vi "Convert Package Attribute Cluster to String.vi"(8 "error in (no error)":errorcluster, 10 "package attributes":T1, 11 "initial package attributes string":string) -> (0 "error out":errorcluster, 3 "package attributes string out":string)   [LabVIEW 2014, in "NIPM_API.lvlib"]
uses:
  NIPM_API.lvlib
  package attributes.ctl
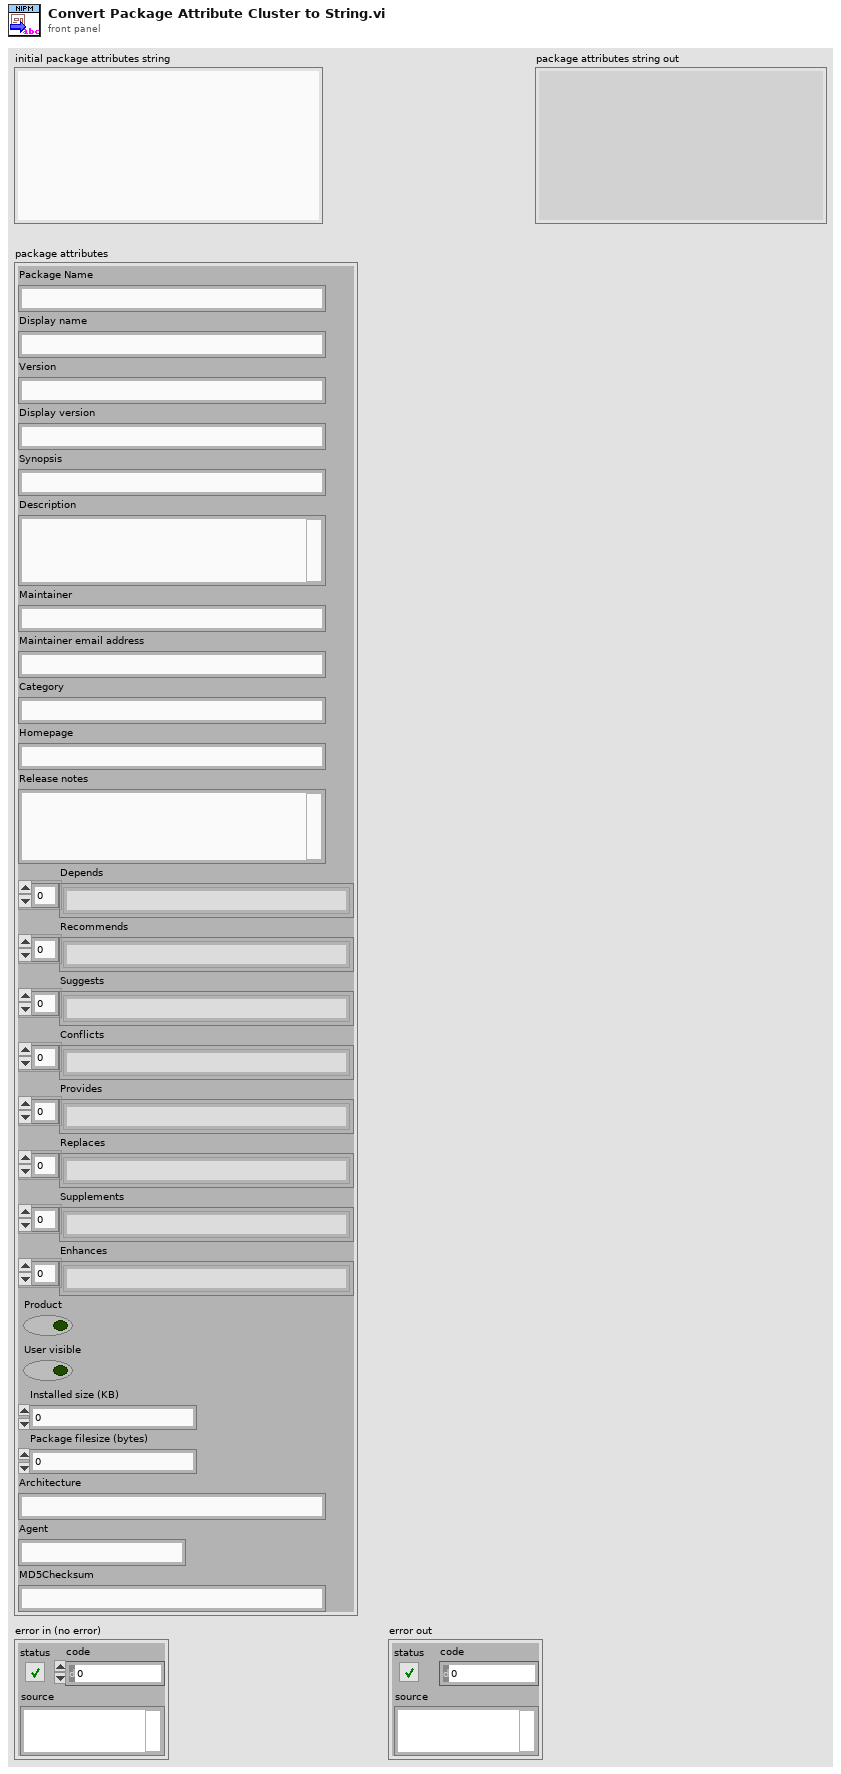
[diagram p1: front panel]
types:
  T1 = typedef "NIPM_API.lvlib/package attributes.ctl" = cluster{"Package Name":string, "Display name":string, "Version":string, "Display version":string, "Synopsis":string, "Description":string, "Maintainer":string, "Maintainer email address":string, "Category":string, "Homepage":string, "Release notes":string, "Depends":string[], "Recommends":string[], "Suggests":string[], "Conflicts":string[], "Provides":string[], "Replaces":string[], "Supplements":string[], "Enhances":string[], "Product":bool, "User visible":bool, "Installed size (KB)":u64, "Package filesize (bytes)":u64, "Architecture":string, "Agent":string, "MD5Checksum":string}
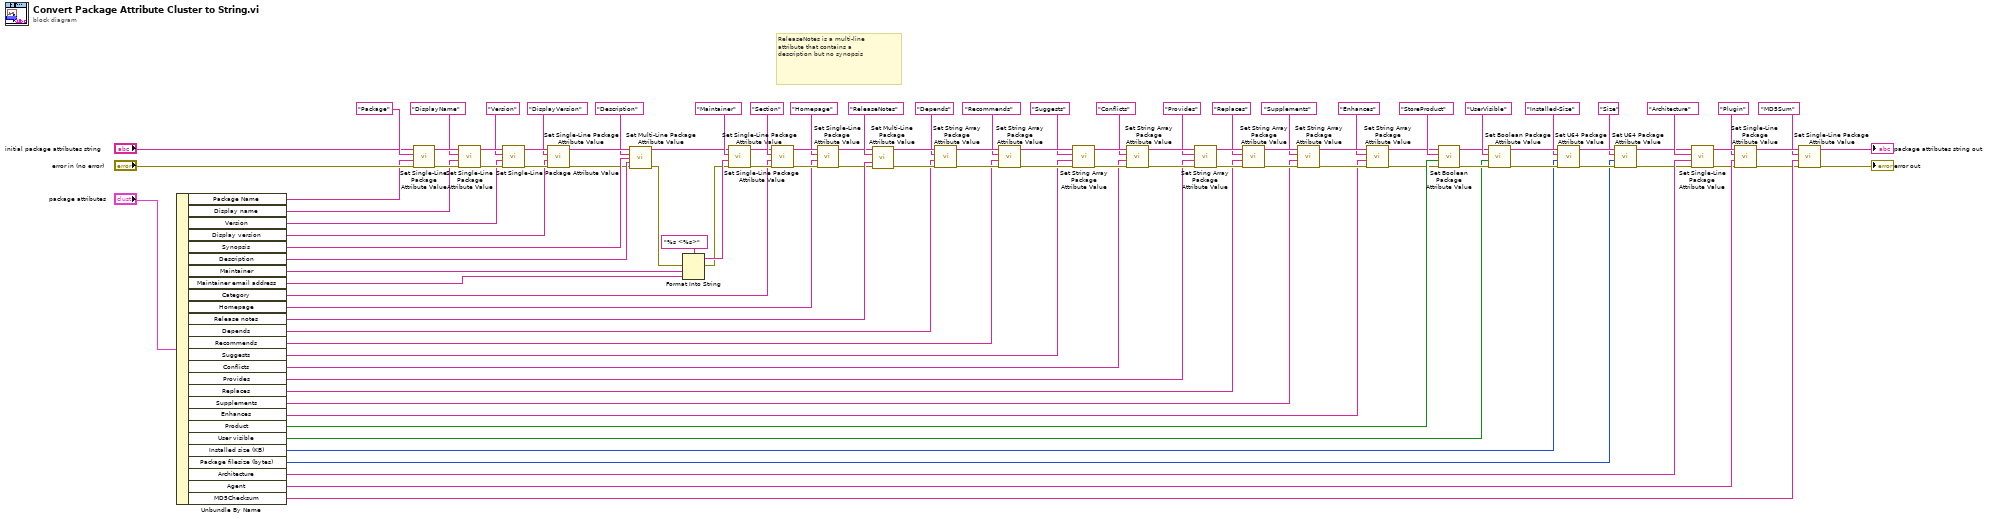
[diagram p0: block diagram]
diagram:
  # "ReleaseNotes is a multi-line attribute that contains a description but no synopsis"
  n1 = Unbundle By Name("package attributes") -> ("Package Name"=w91:string, "Display name"=w90:string, "Version"=w89:string, "Display version"=w88:string, "Synopsis"=w53:string, "Description"=w52:string, "Maintainer"=w69:string, "Maintainer email address"=w68:string, "Category"=w75:string, "Homepage"=w74:string, "Release notes"=w50:string, "Depends"=w20:string[], "Recommends"=w19:string[], "Suggests"=w18:string[], "Conflicts"=w17:string[], "Provides"=w16:string[], "Replaces"=w15:string[], "Supplements"=w14:string[], "Enhances"=w13:string[], "Product"=w60:bool, "User visible"=w59:bool, "Installed size (KB)"=w4:u64, "Package filesize (bytes)"=w3:u64, "Architecture"=w73:string, "Agent"=w72:string, "MD5Checksum"=w71:string)
  n2 = call "Set Single-Line Package Attribute Value.vi"("error in (no error)"="error in (no error)", "package attribute value"=w91, "package attribute name"="Package", "package attributes string in"="initial package attributes string") -> ("error out"=w97:errorcluster, "package attributes string out"=w100:string)  [unwired: 4 in, 2 out]
  n3 = call "Set Single-Line Package Attribute Value.vi"("error in (no error)"=w97, "package attribute value"=w90, "package attribute name"="DisplayName", "package attributes string in"=w100) -> ("error out"=w96:errorcluster, "package attributes string out"=w99:string)  [unwired: 4 in, 2 out]
  n4 = call "Set Single-Line Package Attribute Value.vi"("error in (no error)"=w96, "package attribute value"=w89, "package attribute name"="Version", "package attributes string in"=w99) -> ("error out"=w95:errorcluster, "package attributes string out"=w98:string)  [unwired: 4 in, 2 out]
  n5 = call "Set Single-Line Package Attribute Value.vi"("error in (no error)"=w95, "package attribute value"=w88, "package attribute name"="DisplayVersion", "package attributes string in"=w98) -> ("error out"=w51:errorcluster, "package attributes string out"=w56:string)  [unwired: 4 in, 2 out]
  n6 = call "Set Multi-Line Package Attribute Value.vi"("package attributes string in"=w56, "package attribute name"="Description", "synopsis"=w53, "description"=w52, "error in (no error)"=w51) -> ("package attributes string out"=w55:string, "error out"=w2:errorcluster)  [unwired: 7 in, 2 out]
  n7 = Format Into String(format string="%s <%s>", error in=w2, w69, w68) -> (resulting string=w70:string, error out=w1:errorcluster)  [unwired: 1 in]
  n8 = call "Set Single-Line Package Attribute Value.vi"("error in (no error)"=w1, "package attribute value"=w70, "package attribute name"="Maintainer", "package attributes string in"=w55) -> ("error out"=w82:errorcluster, "package attributes string out"=w85:string)  [unwired: 4 in, 2 out]
  n9 = call "Set Single-Line Package Attribute Value.vi"("error in (no error)"=w82, "package attribute value"=w75, "package attribute name"="Section", "package attributes string in"=w85) -> ("error out"=w81:errorcluster, "package attributes string out"=w84:string)  [unwired: 4 in, 2 out]
  n10 = call "Set Single-Line Package Attribute Value.vi"("error in (no error)"=w81, "package attribute value"=w74, "package attribute name"="Homepage", "package attributes string in"=w84) -> ("error out"=w49:errorcluster, "package attributes string out"=w47:string)  [unwired: 4 in, 2 out]
  n11 = call "Set Multi-Line Package Attribute Value.vi"("package attributes string in"=w47, "package attribute name"="ReleaseNotes", "description"=w50, "error in (no error)"=w49) -> ("package attributes string out"=w30:string, "error out"=w32:errorcluster)  [unwired: 8 in, 2 out]
  n12 = call "Set String Array Package Attribute Value.vi"("error in (no error)"=w32, "package attribute value"=w20, "package attribute name"="Depends" ("Package Attribute Name"), "package attributes string in"=w30) -> ("error out"=w46:errorcluster, "package attributes string out"=w45:string)  [unwired: 4 in, 2 out]
  n13 = call "Set String Array Package Attribute Value.vi"("error in (no error)"=w46, "package attribute value"=w19, "package attribute name"="Recommends" ("Package Attribute Name"), "package attributes string in"=w45) -> ("error out"=w44:errorcluster, "package attributes string out"=w43:string)  [unwired: 4 in, 2 out]
  n14 = call "Set String Array Package Attribute Value.vi"("error in (no error)"=w44, "package attribute value"=w18, "package attribute name"="Suggests" ("Package Attribute Name"), "package attributes string in"=w43) -> ("error out"=w42:errorcluster, "package attributes string out"=w41:string)  [unwired: 4 in, 2 out]
  n15 = call "Set String Array Package Attribute Value.vi"("error in (no error)"=w42, "package attribute value"=w17, "package attribute name"="Conflicts" ("Package Attribute Name"), "package attributes string in"=w41) -> ("error out"=w34:errorcluster, "package attributes string out"=w33:string)  [unwired: 4 in, 2 out]
  n16 = call "Set String Array Package Attribute Value.vi"("error in (no error)"=w34, "package attribute value"=w16, "package attribute name"="Provides" ("Package Attribute Name"), "package attributes string in"=w33) -> ("error out"=w35:errorcluster, "package attributes string out"=w36:string)  [unwired: 4 in, 2 out]
  n17 = call "Set String Array Package Attribute Value.vi"("error in (no error)"=w35, "package attribute value"=w15, "package attribute name"="Replaces" ("Package Attribute Name"), "package attributes string in"=w36) -> ("error out"=w37:errorcluster, "package attributes string out"=w38:string)  [unwired: 4 in, 2 out]
  n18 = call "Set String Array Package Attribute Value.vi"("error in (no error)"=w37, "package attribute value"=w14, "package attribute name"="Supplements" ("Package Attribute Name"), "package attributes string in"=w38) -> ("error out"=w39:errorcluster, "package attributes string out"=w40:string)  [unwired: 4 in, 2 out]
  n19 = call "Set String Array Package Attribute Value.vi"("error in (no error)"=w39, "package attribute value"=w13, "package attribute name"="Enhances" ("Package Attribute Name"), "package attributes string in"=w40) -> ("error out"=w31:errorcluster, "package attributes string out"=w29:string)  [unwired: 4 in, 2 out]
  n20 = call "Set Boolean Package Attribute Value.vi"("error in (no error)"=w31, "package attribute value"=w60, "package attribute name"="StoreProduct", "package attributes string in"=w29) -> ("error out"=w61:errorcluster, "package attributes string out"=w62:string)  [unwired: 4 in, 2 out]
  n21 = call "Set Boolean Package Attribute Value.vi"("error in (no error)"=w61, "package attribute value"=w59, "package attribute name"="UserVisible", "package attributes string in"=w62) -> ("error out"=w11:errorcluster, "package attributes string out"=w9:string)  [unwired: 4 in, 2 out]
  n22 = call "Set U64 Package Attribute Value.vi"("error in (no error)"=w11, "package attribute value"=w4, "package attribute name"="Installed-Size" ("Package Attribute Name"), "package attributes string in"=w9) -> ("error out"=w12:errorcluster, "package attributes string out"=w8:string)  [unwired: 4 in, 2 out]
  n23 = call "Set U64 Package Attribute Value.vi"("error in (no error)"=w12, "package attribute value"=w3, "package attribute name"="Size" ("Package Attribute Name"), "package attributes string in"=w8) -> ("error out"=w10:errorcluster, "package attributes string out"=w7:string)  [unwired: 4 in, 2 out]
  n24 = call "Set Single-Line Package Attribute Value.vi"("error in (no error)"=w10, "package attribute value"=w73, "package attribute name"="Architecture", "package attributes string in"=w7) -> ("error out"=w58:errorcluster, "package attributes string out"=w80:string)  [unwired: 4 in, 2 out]
  n25 = call "Set Single-Line Package Attribute Value.vi"("error in (no error)"=w58, "package attribute value"=w72, "package attribute name"="Plugin", "package attributes string in"=w80) -> ("error out"=w57:errorcluster, "package attributes string out"=w79:string)  [unwired: 4 in, 2 out]
  n26 = call "Set Single-Line Package Attribute Value.vi"("error in (no error)"=w57, "package attribute value"=w71, "package attribute name"="MD5Sum", "package attributes string in"=w79) -> ("error out"=→"error out":errorcluster, "package attributes string out"=→"package attributes string out":string)  [unwired: 4 in, 2 out]
